vi "Close.vi"(0 "comm interface in":refnum<class "Pixy Com.lvclass">, 11 "error in":errorcluster) -> (15 "error out":errorcluster)   [LabVIEW 2018, in "Pixy2.lvlib" / "Pixy Com.lvclass"]
uses:
  Pixy Com.lvclass
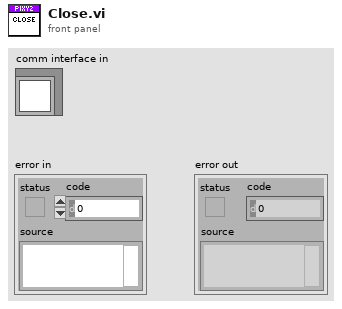
[diagram p1: front panel]
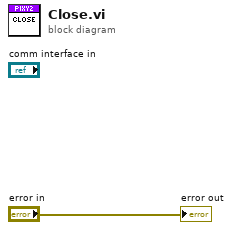
[diagram p0: block diagram]
diagram:
  "error out" <- "error in"
